vi "VS_SetSingleChannel_TS_Step.vi"(0 "Engine reference":refnum<k7>, 5 "Sequence File Ref":refnum<k7>, 7 "Step Name":string="Open Workspace Manager Reference", 9 "Parameter Value array":string[](array[string]), 11 "error in":errorcluster, 12 "Sequence index":i32) -> (4 "Engine reference (out)":refnum<k7>, 6 "Sequence File Ref(out)":refnum<k7>, 15 "error out":errorcluster)   [LabVIEW 2009]
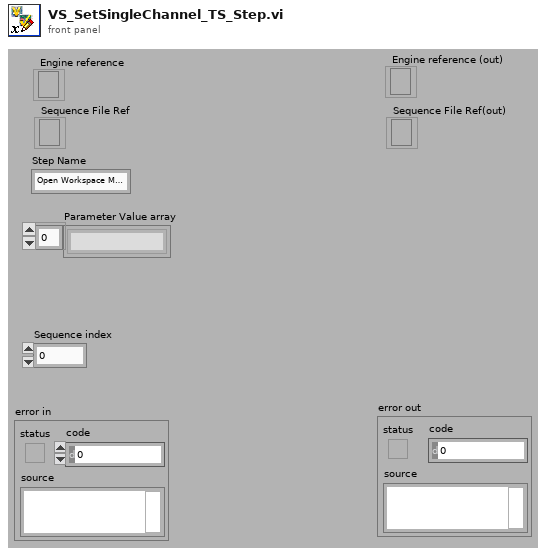
[diagram p1: front panel]
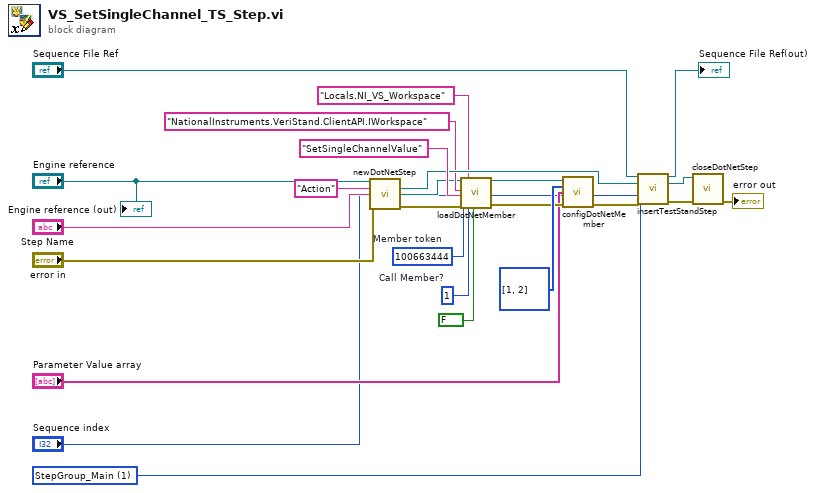
[diagram p0: block diagram]
diagram:
  w23 = 100663444  # Member token
  w21 = 1 items=["StepGroup_Setup", "StepGroup_Main", "StepGroup_Cleanup"] ("Step Group")
  w15 = 1  # Call Member?
  n1 = call "newDotNetStep.vi"("Engine reference"="Engine reference", "stepType"="Action", "Step Name"="Step Name", "error in"="error in") -> ("NewStep (out)"=w20:refnum<k7>, "dotNetModule(out)"=w12:refnum<k7>, "error out"=w24:errorcluster)  [unwired: 8 in, 1 out]
  n2 = call "loadDotNetMember.vi"("dotNetModule"=w12, "ClassName"="NationalInstruments.VeriStand.ClientAPI.IWorkspace", "MemberName"="SetSingleChannelValue", "Member token"=w23, "error in(no error)"=w24, "ClassReference"="Locals.NI_VS_Workspace", "Call Member?"=w15, "CreateObject"=FALSE) -> ("dotNetModule(out)"=w17:refnum<k7>, "error out"=w18:errorcluster)  [unwired: 10 in]
  n3 = call "configDotNetMember.vi"("dotNetModule"=w17, "Index array"=i32[] [1, 2], "Parameter Value array"="Parameter Value array", "error in (no error)"=w18) -> ("error out"=w19:errorcluster)  [unwired: 11 in]
  n4 = call "insertTestStandStep.vi"("Sequence File Ref"="Sequence File Ref", "Step to insert"=w20, "Step Group"=w21, "index"="Sequence index", "error out"=w19) -> ("Sequence File Ref(out)"=→"Sequence File Ref(out)":refnum<k7>, "Step to insert (out)"=w9:refnum<k7>, "error out"=w8:errorcluster)  [unwired: 8 in]
  n5 = call "closeDotNetStep.vi"("error in"=w8, "NewStep"=w9) -> ("error out"=→"error out":errorcluster)  [unwired: 9 in]
  "Engine reference (out)" <- "Engine reference"
